vi "Syntethic data generator.vi"(8 "Error In":errorcluster, 10 "Channel map":u16) -> (0 "Error Out":errorcluster, 2 "Char value":u8[](array[numeric]))   [LabVIEW 2016]
panel:
  out "Channel map (bin)":u16 format="%016b"
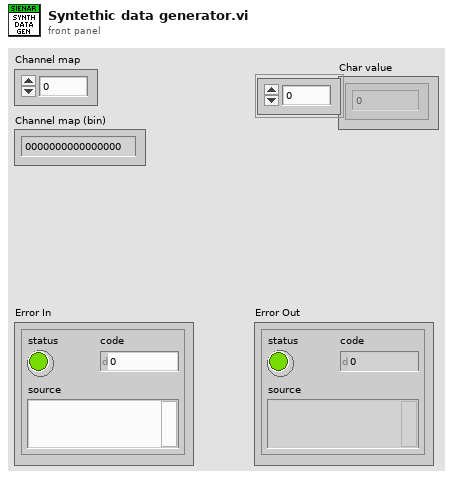
[diagram p1: front panel]
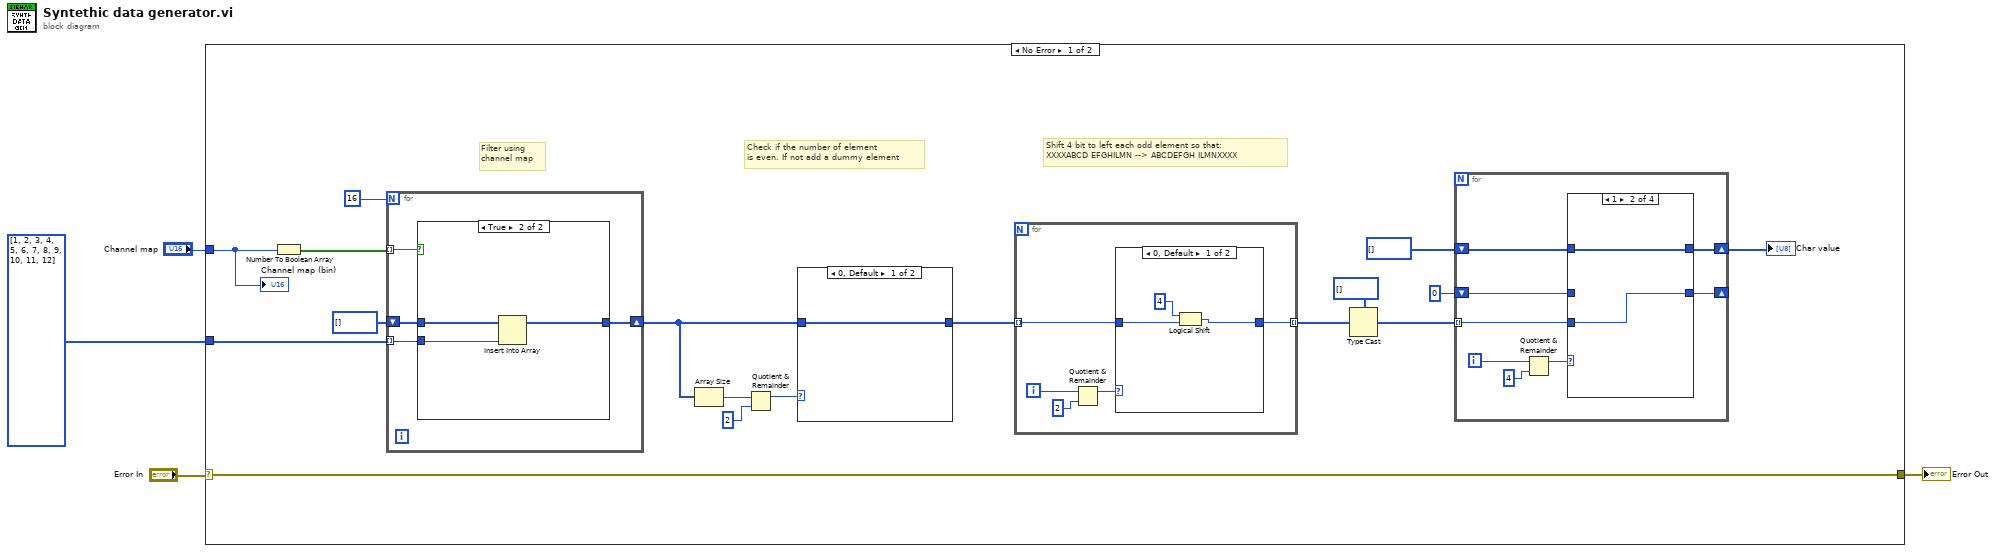
[diagram p0: block diagram]
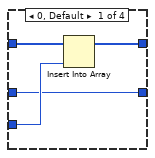
[diagram p2: hidden frame]
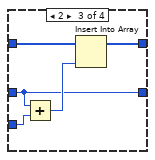
[diagram p3: hidden frame]
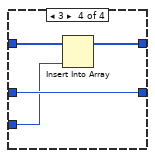
[diagram p4: hidden frame]
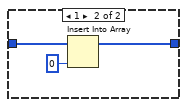
[diagram p6: hidden frame]
diagram:
  n1 = case shown="No Error" "Error In" {
    selector: "Error In" -> [w21 w66]
    tunnel: [w21 w66] -> w3
    tunnel: "Channel map" -> [w20 _]
    tunnel: u16[] [1, 2, 3, 4, 5, 6, 7, 8, 9, 10, 11, 12] -> [w18 _]
    frame No Error {
      # "Shift 4 bit to left each odd element so that:\nXXXXABCD EFGHILMN --> ABCDEFGH ILMNXXXX"
      # "Check if the number of element\nis even. If not add a dummy element"
      # "Filter using \nchannel map"
      n2 = Number To Boolean Array(number=w20) -> (Boolean array=w19:bool[])
      n3 = for {
        N: 16 -> [_]
        tunnel: w19 -> [w61] mode=indexing
        tunnel: w18 -> [w60] mode=indexing
        shift-right: [w59] -> w12
        shift-left: u16[] [] -> [w58]
        n4 = case shown="True" w61 {
          tunnel: w60 -> [_ w65]
          tunnel: [w62 w64] -> w59
          tunnel: w58 -> [w62 w63]
          frame False {
          }
          frame True {
            n5 = Insert Into Array(array=w63, new element=w65) -> (w64:u16[])  [unwired: 1 in]
          }
        }
      }
      n6 = Array Size(array=w12) -> (size(s)=w15:i32)
      n7 = Quotient & Remainder(x=w15, y=2) -> (x-y*floor(x/y)=w14:i32)  [unwired: 1 out]
      n8 = case shown="0, Default" w14 {
        tunnel: w12 -> [w54 w57]
        tunnel: [w54 w55] -> w11
        frame 0, Default {
        }
        frame 1 {
          n9 = Insert Into Array(array=w57, new element=u16 0 ("new element/subarray")) -> (w55:u16[])  [unwired: 1 in]
        }
      }
      n10 = for {
        tunnel: w11 -> [w46] mode=indexing
        tunnel: [w45] -> w10 mode=indexing
        i -> [w48]
        n11 = Quotient & Remainder(x=w48, y=2) -> (x-y*floor(x/y)=w47:i32)  [unwired: 1 out]
        n12 = case shown="0, Default" w47 {
          tunnel: w46 -> [w51 w53]
          tunnel: [w50 w53] -> w45
          frame 0, Default {
            n13 = Logical Shift(y=i16 4, x=w51) -> (x << y=w50:u16)
          }
          frame 1 {
          }
        }
      }
      n14 = Type Cast(type=u8[] [], x=w10) -> (*(type *) &x=w8:u8[])
      n15 = for {
        tunnel: w8 -> [w26] mode=indexing
        shift-right: [w24] -> w5
        shift-left: u8[] [] -> [w25]
        shift-right: [w23] -> _
        shift-left: u8 0 -> [w22]
        i -> [w28]
        n16 = Quotient & Remainder(x=w28, y=4) -> (x-y*floor(x/y)=w27:i32)  [unwired: 1 out]
        n17 = case shown="1" w27 {
          tunnel: w26 -> [w33 w34 w38 w41]
          tunnel: w25 -> [w32 w35 w39 w44]
          tunnel: [w31 w35 w40 w43] -> w24
          tunnel: [w30 w34 w36 w42] -> w23
          tunnel: w22 -> [w30 _ w36 w42]
          frame 0, Default {
            n18 = Insert Into Array(array=w32, new element=w33) -> (w31:u8[])  [unwired: 1 in]
          }
          frame 1 {
          }
          frame 2 {
            n19 = Add(x=w36, y=w38) -> (x+y=w37:u8)
            n20 = Insert Into Array(array=w39, new element=w37) -> (w40:u8[])  [unwired: 1 in]
          }
          frame 3 {
            n21 = Insert Into Array(array=w44, new element=w41) -> (w43:u8[])  [unwired: 1 in]
          }
        }
      }
      "Char value" <- w5
      "Channel map (bin)" <- w20
    }
    frame Error {
    }
  }
  "Error Out" <- w3
